vi "Main.vi"() -> ()   [LabVIEW 2015]
doc: "The myRIO Project template acquires acceleration data from the onboard accelerometer and displays the changes of acceleration values in a waveform chart."
panel:
  in  "Boolean":bool
  out "Phrase":string
  out "Word":string
  out "Symbols":string
  out "Time":dbl
  in  "stop":bool
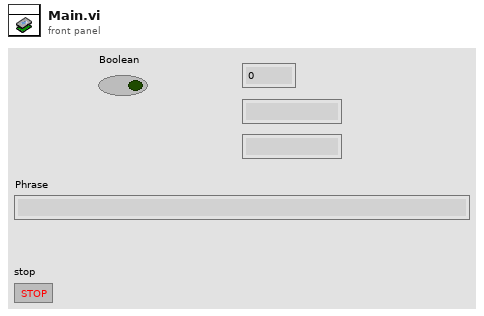
[diagram p1: front panel]
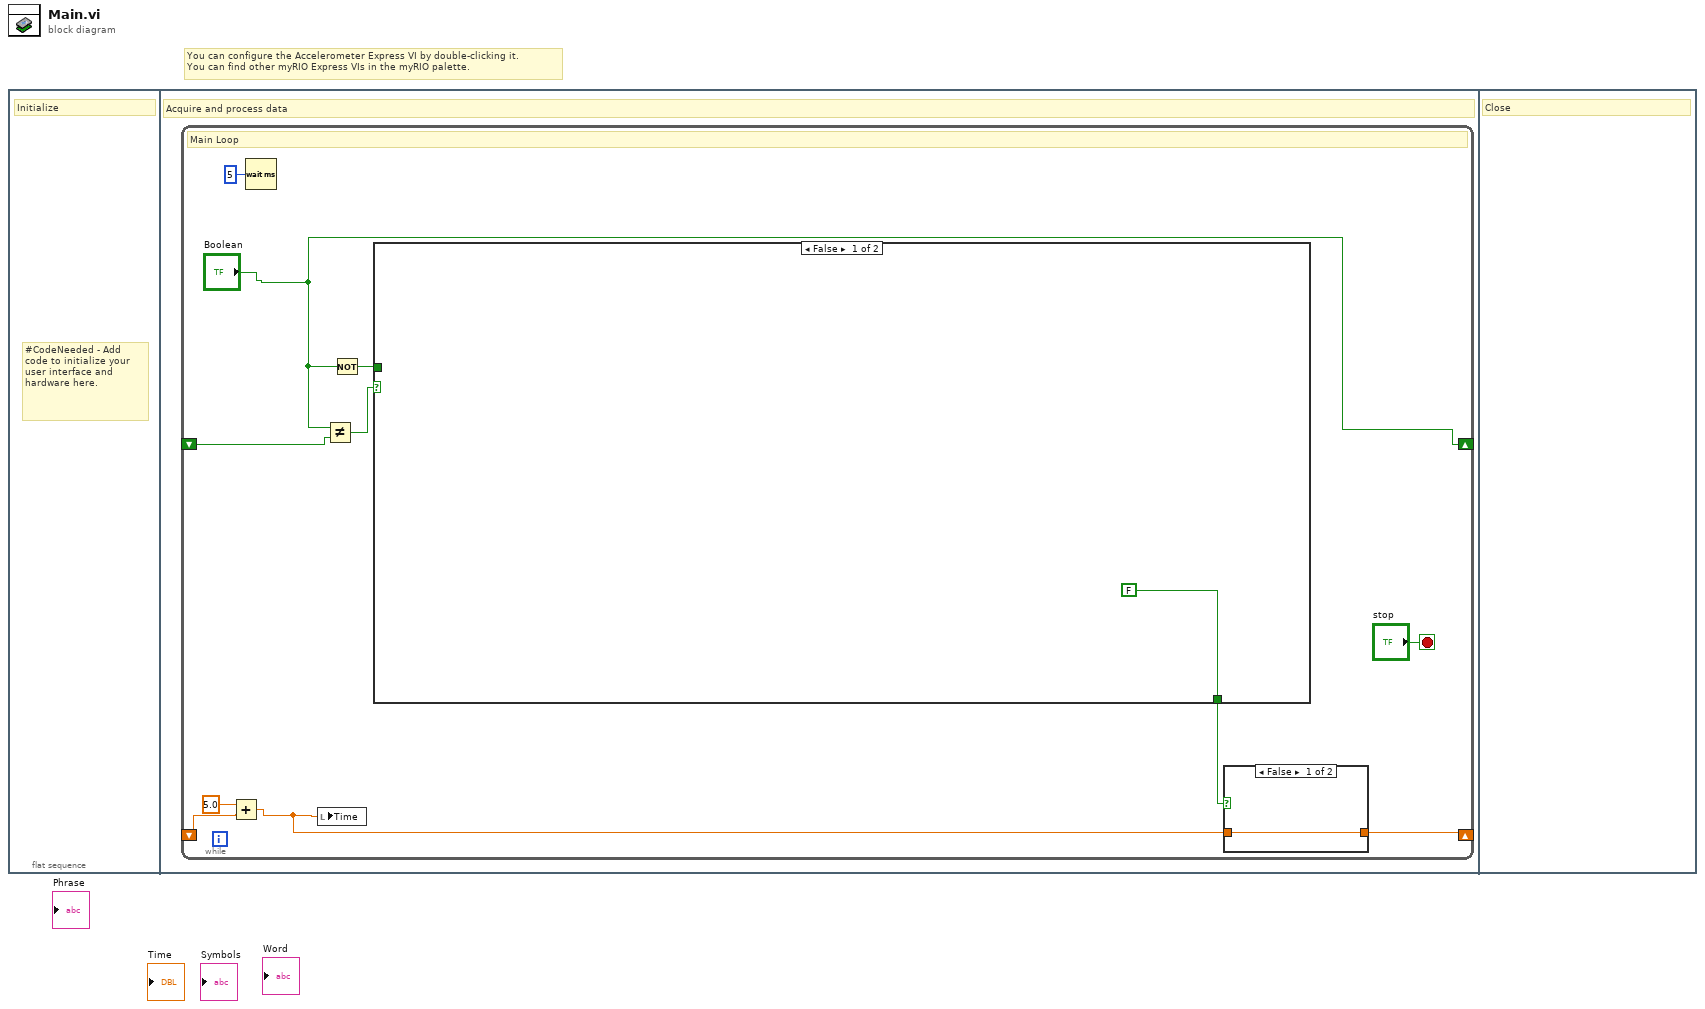
[diagram p0: block diagram]
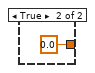
[diagram p2: hidden frame]
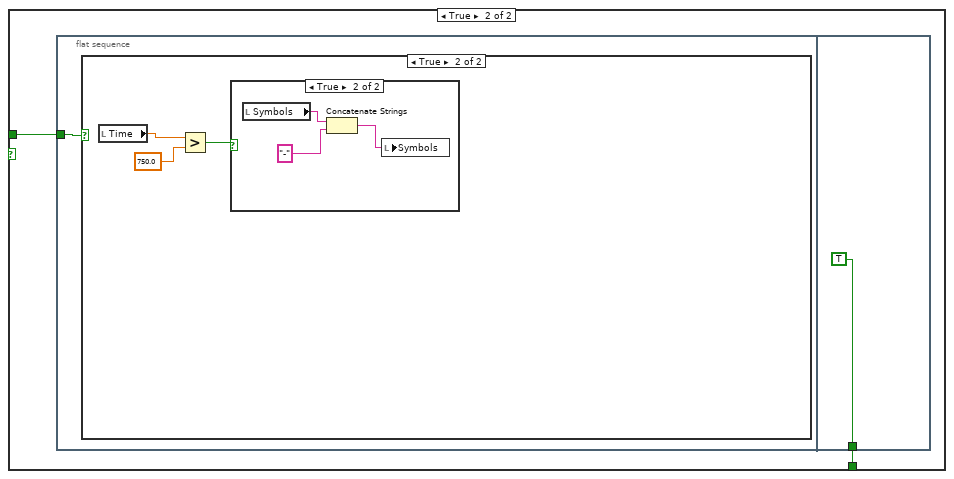
[diagram p3: hidden frame]
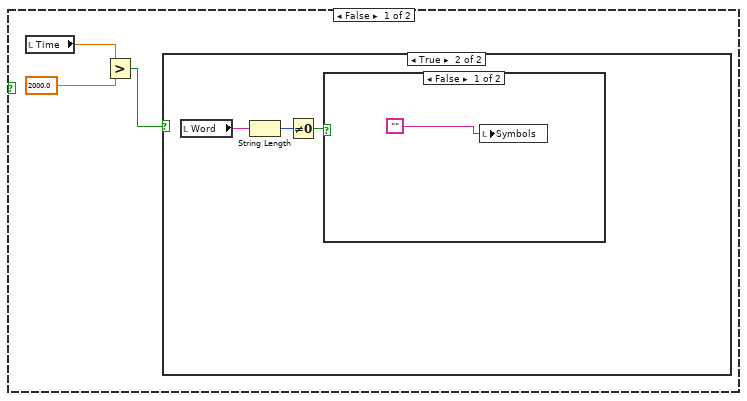
[diagram p4: hidden frame]
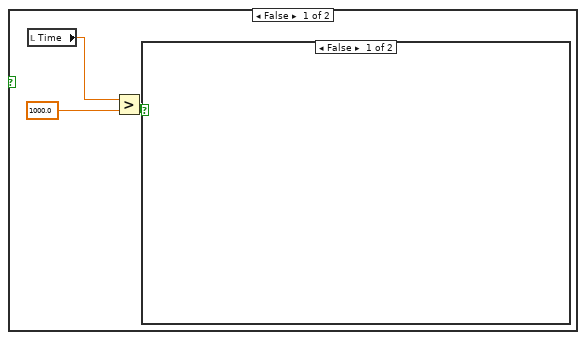
[diagram p5: hidden frame]
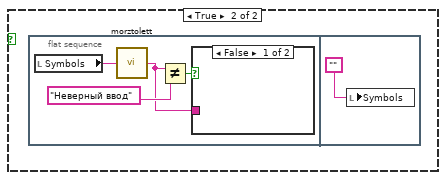
[diagram p6: hidden frame]
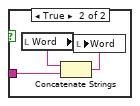
[diagram p7: hidden frame]
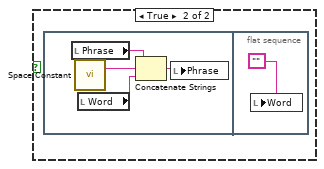
[diagram p8: hidden frame]
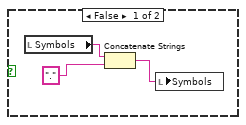
[diagram p9: hidden frame]
diagram:
  # "You can configure the Accelerometer Express VI by double-clicking it.\nYou can find other myRIO Express VIs in the myRIO palette."
  n1 = flat-sequence {
    frame #0 {
      # "#CodeNeeded - Add code to initialize your user interface and hardware here."
      # "Initialize"
    }
    frame #1 {
      # "Acquire and process data"
      n2 = while {
        shift-right: [w1] -> _
        shift-left: _ -> [w5]
        shift-right: ["Boolean"] -> _
        shift-left: _ -> [w9]
        stop <- "stop" stop-if-true
        # "Main Loop"
        n3 = Add(x=5.0, y=w5) -> (x+y=w2:dbl)
        n4 = Wait (ms)(milliseconds to wait=u32 5) -> ()  [unwired: 1 out]
        n5 = local write "Time"(w2) -> ()
        n6 = Not Equal?(x="Boolean", y=w9) -> (x != y?=w8:bool)
        n7 = Not(x="Boolean") -> (.not. x?=w7:bool)
        n8 = case shown="False" w8 {
          tunnel: w7 -> [_ w16]
          tunnel: [FALSE w15] -> w3
          frame False {
          }
          frame True {
            n9 = flat-sequence {
              tunnel: w16 -> [w17]
              tunnel: [TRUE] -> w15
              frame #0 {
                n10 = case shown="True" w17 {
                  frame False {
                    n11 = local read "Time"() -> (w20:dbl)
                    n12 = Greater?(x=w20, y=2000.0) -> (0:w18:bool)
                    n13 = case shown="True" w18 {
                      frame False {
                        n14 = local read "Time"() -> (w22:dbl)
                        n15 = Greater?(x=w22, y=1000.0) -> (0:w21:bool)
                        n16 = case shown="False" w21 {
                          frame False {
                          }
                          frame True {
                            n17 = flat-sequence {
                              frame #0 {
                                n18 = local read "Symbols"() -> (w25:string)
                                n19 = call "morztolett.vi"("String"=w25) -> ("String 2"=w24:string)
                                n20 = Not Equal?(x=w24, y="Неверный ввод") -> (x != y?=w27:bool)
                                n21 = case shown="False" w27 {
                                tunnel: w24 -> [_ w29]
                                frame False {
                                }
                                frame True {
                                n22 = local read "Word"() -> (w30:string)
                                n23 = Concatenate Strings(w30, w29) -> (w28:string)
                                n24 = local write "Word"(w28) -> ()
                                }
                                }
                              }
                              frame #1 {
                                n25 = local write "Symbols"("") -> ()
                              }
                            }
                          }
                        }
                      }
                      frame True {
                        n26 = local read "Word"() -> (w33:string)
                        n27 = String Length(string=w33) -> (length=w34:i32)
                        n28 = Not Equal To 0?(x=w34) -> (x != 0?=w32:bool)
                        n29 = case shown="False" w32 {
                          frame False {
                            n30 = local write "Symbols"("") -> ()
                          }
                          frame True {
                            n31 = flat-sequence {
                              frame #0 {
                                n32 = local read "Phrase"() -> (w37:string)
                                n33 = call <vilib>:"Space Constant.vi"() -> ("String"=w36:string)
                                n34 = local read "Word"() -> (w38:string)
                                n35 = Concatenate Strings(w37, w36, w38) -> (w39:string)
                                n36 = local write "Phrase"(w39) -> ()
                              }
                              frame #1 {
                                n37 = local write "Word"("") -> ()
                              }
                            }
                          }
                        }
                      }
                    }
                  }
                  frame True {
                    n38 = local read "Time"() -> (w43:dbl)
                    n39 = Greater?(x=w43, y=750.0) -> (0:w41:bool)
                    n40 = case shown="True" w41 {
                      frame False {
                        n41 = local read "Symbols"() -> (w46:string)
                        n42 = Concatenate Strings(w46, ".") -> (w45:string)
                        n43 = local write "Symbols"(w45) -> ()
                      }
                      frame True {
                        n44 = local read "Symbols"() -> (w48:string)
                        n45 = Concatenate Strings(w48, "-") -> (w47:string)
                        n46 = local write "Symbols"(w47) -> ()
                      }
                    }
                  }
                }
              }
              frame #1 {
              }
            }
          }
        }
        n47 = case shown="False" w3 {
          tunnel: w2 -> [w12 _]
          tunnel: [w12 0.0] -> w1
          frame False {
          }
          frame True {
          }
        }
      }
    }
    frame #2 {
      # "Close"
    }
  }
